vi "Load Patterns.vi"(8 "error in (no error)":errorcluster, 11 "instrument handle":refnum<k15>) -> (0 "error out":errorcluster, 3 "instrument handle out":refnum<k15>)   [LabVIEW 2018]
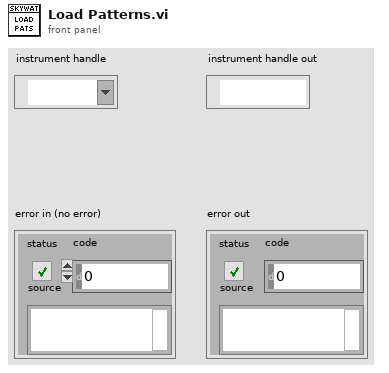
[diagram p1: front panel]
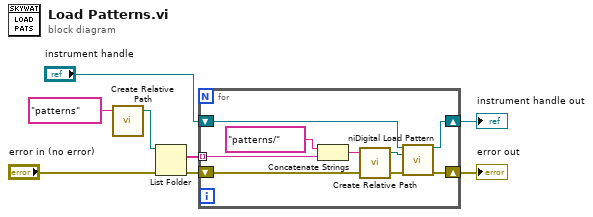
[diagram p0: block diagram]
diagram:
  n1 = call "Create Relative Path.vi"("file name"="patterns" ("string")) -> ("appended path"=w1:path)  [unwired: 4 in]
  n2 = List Folder(path=w1, error in="error in (no error)") -> (filenames=w5:string[], error out=w3:errorcluster)  [unwired: 2 in, 2 out]
  n3 = for {
    tunnel: w5 -> [w14] mode=indexing
    shift-right: [w11] -> w7
    shift-left: "instrument handle" -> [w12]
    shift-right: [w10] -> w6
    shift-left: w3 -> [w9]
    n4 = Concatenate Strings("patterns/" ("string"), w14) -> (w13:string)
    n5 = call "Create Relative Path.vi"("file name"=w13) -> ("appended path"=w16:path)  [unwired: 4 in]
    n6 = call <instrlib>:"niDigital Load Pattern.vi"("instrument handle"=w12, "pattern file"=w16, "error in"=w9) -> ("instrument handle out"=w11:refnum<k15>, "error out"=w10:errorcluster)  [unwired: 11 in]
  }
  "instrument handle out" <- w7
  "error out" <- w6
